vi "Demo(冲突时的文件备份2013-03-27 14-06-05).vi"() -> ()   [LabVIEW 2012, in "DriveInfo.lvclass"]
uses:
  DriveInfo.lvclass
  Info.ctl
panel:
  out "Drives":T1[](array[typedef]) {"DriveType" items=["Unknown", "NoRootDirectory", "Removable", "Fixed", "Network", "CDRom", "Ram"]}
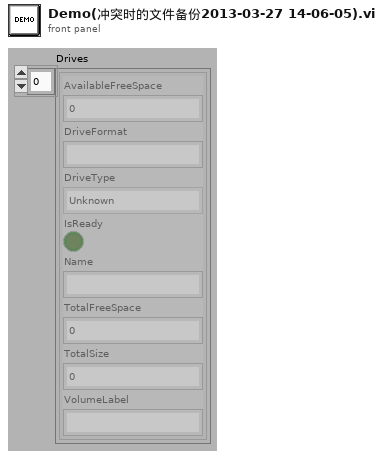
[diagram p1: front panel]
types:
  T1 = typedef "DriveInfo.lvclass/Info.ctl" = cluster{"AvailableFreeSpace":i64, "DriveFormat":string, "DriveType":i32, "IsReady":bool, "Name":string, "TotalFreeSpace":i64, "TotalSize":i64, "VolumeLabel":string}
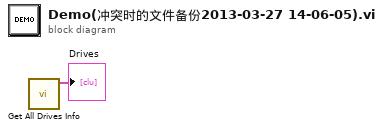
[diagram p0: block diagram]
diagram:
  n1 = call "Get All Drives Info.vi"() -> ("Drives"=→"Drives":T1[])  [unwired: 10 in, 1 out]
